vi "increment filename.vi"(1 "path":path=path "C:/user/patrick/test/test/filename.itx") -> (0 "modified path":path=path "C:/")   [LabVIEW 2013]
uses:
  FilePath.glb.vi
panel:
  out "Numeric":i32
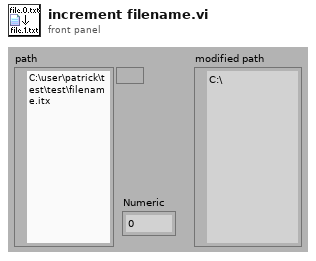
[diagram p1: front panel]
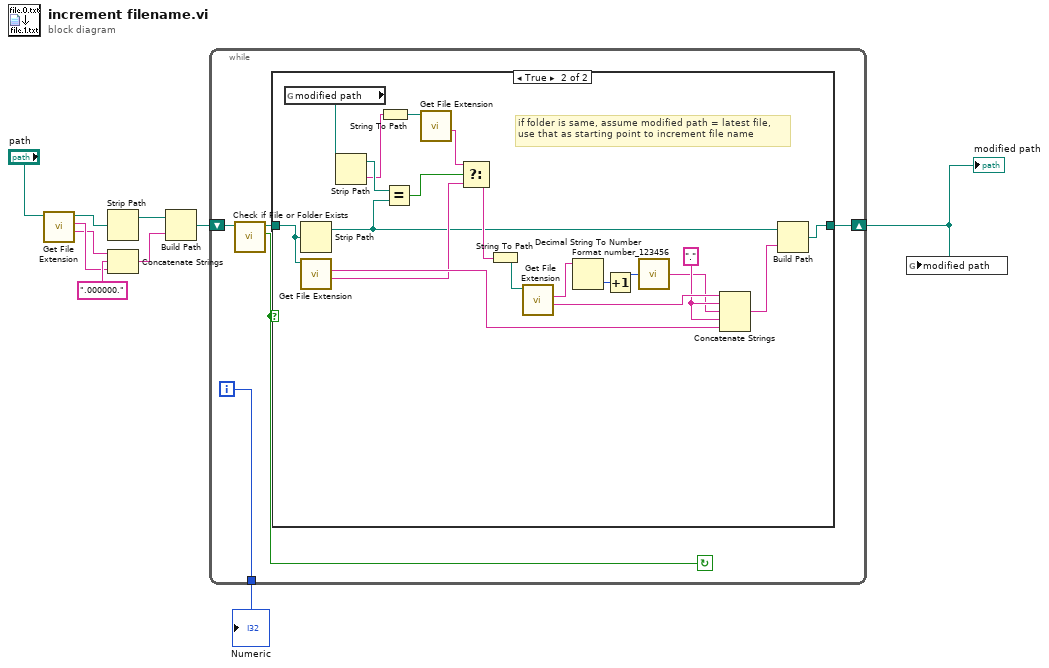
[diagram p0: block diagram]
diagram:
  n1 = call <vilib>:"Get File Extension.vi"("file"="path") -> ("filename without extension"=w8:string, "lowercase file extension"=w9:string, "dup file"=w5:path)  [unwired: 1 in, 7 out]
  n2 = Strip Path(path=w5) -> (stripped path=w4:path)  [unwired: 1 out]
  n3 = Concatenate Strings(w8, ".000000.", w9) -> (w3:string)
  n4 = Build Path(base path=w4, name or relative path=w3) -> (appended path=w7:path)
  n5 = while {
    shift-right: [w11] -> w1
    shift-left: w7 -> [w14]
    tunnel: [w12] -> w2
    i -> [w12]
    stop <- w13 continue-if-true
    n6 = call <vilib>:"Check if File or Folder Exists.vi"("path"=w14) -> ("file or folder exists?"=w13:bool, "dup path"=w15:path)  [unwired: 1 in, 8 out]
    n7 = case shown="True" w13 {
      tunnel: w15 -> [w16 w36]
      tunnel: [w16 w35] -> w11
      frame False {
      }
      frame True {
        w29 = "." ("regular expression")
        # "if folder is same, assume modified path = latest file,\nuse that as starting point to increment file name"
        n8 = global read "FilePath.glb.vi" "modified path"() -> (w17:path)
        n9 = Strip Path(path=w36) -> (stripped path=w23:path)  [unwired: 1 out]
        n10 = call <vilib>:"Get File Extension.vi"("file"=w36) -> ("filename without extension"=w24:string, "lowercase file extension"=w34:string)  [unwired: 1 in, 8 out]
        n11 = Strip Path(path=w17) -> (stripped path=w21:path, name=w18:string)
        n12 = String To Path(string=w18) -> (path=w22:path)
        n13 = Equal?(x=w21, y=w23) -> (x = y?=w20:bool)
        n14 = call <vilib>:"Get File Extension.vi"("file"=w22) -> ("filename without extension"=w19:string)  [unwired: 1 in, 9 out]
        n15 = Select(t=w19, s=w20, f=w24) -> (s? t:f=w25:string)
        n16 = String To Path(string=w25) -> (path=w32:path)
        n17 = call <vilib>:"Get File Extension.vi"("file"=w32) -> ("filename without extension"=w30:string, "lowercase file extension"=w31:string)  [unwired: 1 in, 8 out]
        n18 = Decimal String To Number(string=w31) -> (number=w26:i32)  [unwired: 1 in, 2 out]
        n19 = Increment(x=w26) -> (x+1=w27:i32)
        n20 = call <userlib>:"Format number_123456.vi"("number"=w27) -> ("String"=w28:string)
        n21 = Concatenate Strings(w30, w29, w28, w29, w34) -> (w33:string)
        n22 = Build Path(base path=w23, name or relative path=w33) -> (appended path=w35:path)
      }
    }
  }
  "modified path" <- w1
  "Numeric" <- w2
  n23 = global write "FilePath.glb.vi" "modified path"(w1) -> ()
